vi "TestDurarion.vi"() -> ()   [LabVIEW 2015]
panel:
  out "concatenated string":string
  in  "Stop Button":bool
  out "Time elapsed":dbl
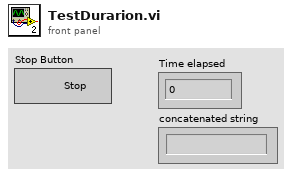
[diagram p1: front panel]
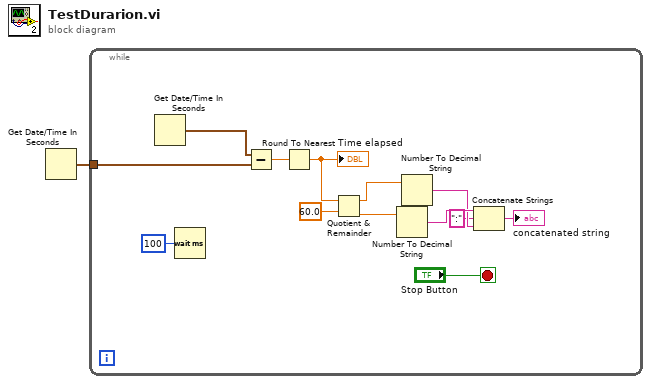
[diagram p0: block diagram]
diagram:
  n1 = Get Date/Time In Seconds() -> (seconds since 1Jan1904=w1:timestamp)
  n2 = while {
    tunnel: w1 -> [w13]
    stop <- "Stop Button" stop-if-true
    n3 = Get Date/Time In Seconds() -> (seconds since 1Jan1904=w14:timestamp)
    n4 = Wait (ms)(milliseconds to wait=u32 100) -> ()  [unwired: 1 out]
    n5 = Subtract(x=w14, y=w13) -> (x-y=w10:dbl)
    n6 = Round To Nearest(number=w10) -> (nearest integer value=w9:dbl)
    "Time elapsed" <- w9
    n7 = Quotient & Remainder(x=w9, y=60.0) -> (x-y*floor(x/y)=w6:dbl, floor(x/y)=w7:dbl)
    n8 = Number To Decimal String(number=w7) -> (decimal integer string=w5:string)  [unwired: 1 in]
    n9 = Number To Decimal String(number=w6) -> (decimal integer string=w4:string)  [unwired: 1 in]
    n10 = Concatenate Strings(w5, ":" ("string"), w4) -> (→"concatenated string":string)
  }
